vi "Disconnect Channels (Single).vi"(8 "error in (no error)":errorcluster, 9 "channel 2":string, 10 "channel 1":string, 11 "SLSC Switch in":refnum<class "SLSC Switch.lvclass">) -> (0 "error out":errorcluster, 3 "SLSC Switch out":refnum<class "SLSC Switch.lvclass">)   [LabVIEW 2016, in "SLSC Switch.lvlib" / "SLSC Switch.lvclass"]
doc: "Breaks the path between two channels created with the Connect Channels VI. If no connection exists between the channels, SLSC-SWITCH returns an error."
uses:
  SLSC Switch.lvclass
  SLSC Switch.lvclass/SLSC Switch.ctl
  slscsl/slscsl.lvclass
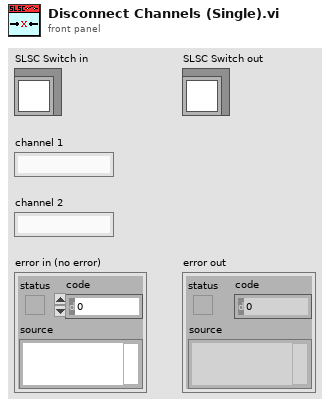
[diagram p1: front panel]
types:
  T1 = typedef "SLSC Switch.lvlib/slscsl.lvclass/SwitchActionsArray.ctl" = T2[]
  T2 = typedef "SLSC Switch.lvlib/slscsl.lvclass/SwitchAction.ctl" = cluster{"index":i32, "RelayAction":T3}
  T3 = typedef "SLSC Switch.lvlib/slscsl.lvclass/RelayAction.ctl" = u32
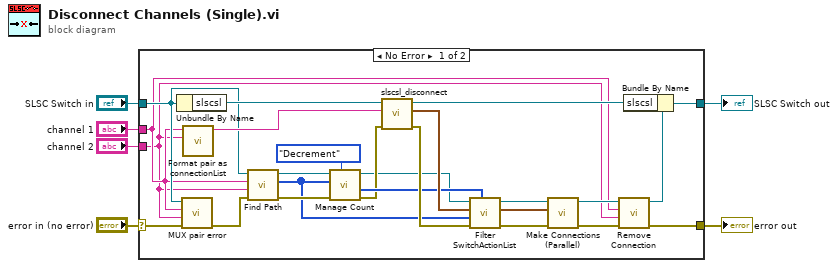
[diagram p0: block diagram]
diagram:
  n1 = case shown="No Error" "error in (no error)" {
    selector: "error in (no error)" -> [w26 w33]
    tunnel: [w7 w33] -> w5
    tunnel: "channel 1" -> [w24 _]
    tunnel: "channel 2" -> [w23 _]
    tunnel: [w8 w32] -> w2
    tunnel: "SLSC Switch in" -> [w25 w32]
    frame No Error {
      n2 = Unbundle By Name(w25) -> ("slscsl"=w31:refnum<class "slscsl.lvclass">)
      n3 = call "MUX pair error.vi"("error in (no error)"=w26, "channel 2"=w23, "channel 1"=w24, "SLSC Switch in"=w25) -> ("error out"=w22:errorcluster)  [unwired: 7 in]
      n4 = call "Format pair as connectionList.vi"("channel in"=w23, "channel 1"=w24) -> ("connectionList"=w30:string)  [unwired: 9 in]
      n5 = call "Find Path.vi"("error in (no error)"=w22, "channel 2"=w23, "channel 1"=w24, "SLSC Switch in"=w25) -> ("error out"=w14:errorcluster, "Relay Indexes"=w10:i32[], "SLSC Switch out"=w12:refnum<class "SLSC Switch.lvclass">)  [unwired: 5 in]
      n6 = call "Manage Count.vi"("Inc/Dec"=enum16{"Increment", "Decrement"}."Decrement", "error in (no error)"=w14, "Relay Indexes"=w10, "SLSC Switch in"=w12) -> ("error out"=w13:errorcluster, "Relay Counts"=w15:i32[], "SLSC Switch out"=w11:refnum<class "SLSC Switch.lvclass">)  [unwired: 5 in]
      n7 = call "slscsl_disconnect.vi"("error in (no error)"=w13, "connectionList"=w30, "slscsl in"=w31) -> ("error out"=w18:errorcluster, "SwitchActionsArray"=w21:T1, "slscsl out"=w27:refnum<class "slscsl.lvclass">)  [unwired: 6 in]
      n8 = call "Filter SwitchActionList.vi"("Relay Counts"=w15, "error in (no error)"=w18, "Relay Indexes"=w10, "SwitchActionList in"=w21, "SLSC Switch in"=w11) -> ("error out"=w17:errorcluster, "SwitchActionList out"=w20:T1, "SLSC Switch out"=w19:refnum<class "SLSC Switch.lvclass">)  [unwired: 4 in]
      n9 = call "Make Connections (Parallel).vi"("error in (no error)"=w17, "switchActionsArray"=w20, "SLSC Switch in"=w19) -> ("error out"=w29:errorcluster, "SLSC Switch out"=w28:refnum<class "SLSC Switch.lvclass">)  [unwired: 7 in]
      n10 = call "Remove Connection.vi"("error in (no error)"=w29, "channel 2"=w23, "channel 1"=w24, "SLSC Switch in"=w28) -> ("error out"=w7:errorcluster, "SLSC Switch out"=w9:refnum<class "SLSC Switch.lvclass">)  [unwired: 6 in]
      n11 = Bundle By Name(cluster=w9, "slscsl"=w27) -> (w8:refnum<class "SLSC Switch.lvclass">)
    }
    frame Error {
    }
  }
  "error out" <- w5
  "SLSC Switch out" <- w2
